vi "Upload info from spreadsheet.vi"(11 "Upload Spreadsheet path":path) -> (3 "Cell Settings Array 1":T1(array[cluster])=[{"Cell Position"=1, "Cell Label"="", "Pixel to measure"=0, "Area (cm^2)"=0.126, "Variable"="", "Variable value"="", "Scan settings in queue"=0}, {"Cell Position"=2, "Cell Label"="", "Pixel to measure"=0, "Area (cm^2)"=0.126, "Variable"="", "Variable value"="", "Scan settings in queue"=0}, {"Cell Position"=3, "Cell Label"="", "Pixel to measure"=0, "Area (cm^2)"=0.126, "Variable"="", "Variable value"="", "Scan settings in queue"=0}, {"Cell Position"=4, "Cell Label"="", "Pixel to measure"=0, "Area (cm^2)"=0.126, "Variable"="", "Variable value"="", "Scan settings in queue"=0}, {"Cell Position"=5, "Cell Label"="", "Pixel to measure"=0, "Area (cm^2)"=0.126, "Variable"="", "Variable value"="", "Scan settings in queue"=0}, {"Cell Position"=6, "Cell Label"="", "Pixel to measure"=0, "Area (cm^2)"=0.126, "Variable"="", "Variable value"="", "Scan settings in queue"=0}, {"Cell Position"=7, "Cell Label"="", "Pixel to measure"=0, "Area (cm^2)"=0.126, "Variable"="", "Variable value"="", "Scan settings in queue"=0}, {"Cell Position"=8, "Cell Label"="", "Pixel to measure"=0, "Area (cm^2)"=0.126, "Variable"="", "Variable value"="", "Scan settings in queue"=0}, {"Cell Position"=9, "Cell Label"="", "Pixel to measure"=0, "Area (cm^2)"=0.126, "Variable"="", "Variable value"="", "Scan settings in queue"=0}, {"Cell Position"=10, "Cell Label"="", "Pixel to measure"=0, "Area (cm^2)"=0.126, "Variable"="", "Variable value"="", "Scan settings in queue"=0}, {"Cell Position"=11, "Cell Label"="", "Pixel to measure"=0, "Area (cm^2)"=0.126, "Variable"="", "Variable value"="", "Scan settings in queue"=0}, {"Cell Position"=12, "Cell Label"="", "Pixel to measure"=0, "Area (cm^2)"=0.126, "Variable"="", "Variable value"="", "Scan settings in queue"=0}, {"Cell Position"=13, "Cell Label"="", "Pixel to measure"=0, "Area (cm^2)"=0.126, "Variable"="", "Variable value"="", "Scan settings in queue"=0}, {"Cell Position"=14, "Cell Label"="", "Pixel to measure"=0, "Area (cm^2)"=0.126, "Variable"="", "Variable value"="", "Scan settings in queue"=0}, {"Cell Position"=15, "Cell Label"="", "Pixel to measure"=0, "Area (cm^2)"=0.126, "Variable"="", "Variable value"="", "Scan settings in queue"=0}, {"Cell Position"=16, "Cell Label"="", "Pixel to measure"=0, "Area (cm^2)"=0.126, "Variable"="", "Variable value"="", "Scan settings in queue"=0}] {"Pixel to measure" items=["All", "1", "2", "3", "4", "5", "6", "7", "8"]})   [LabVIEW 2011]
uses:
  <vilib>/Utility/file.llb/Read From Spreadsheet File (string).vi
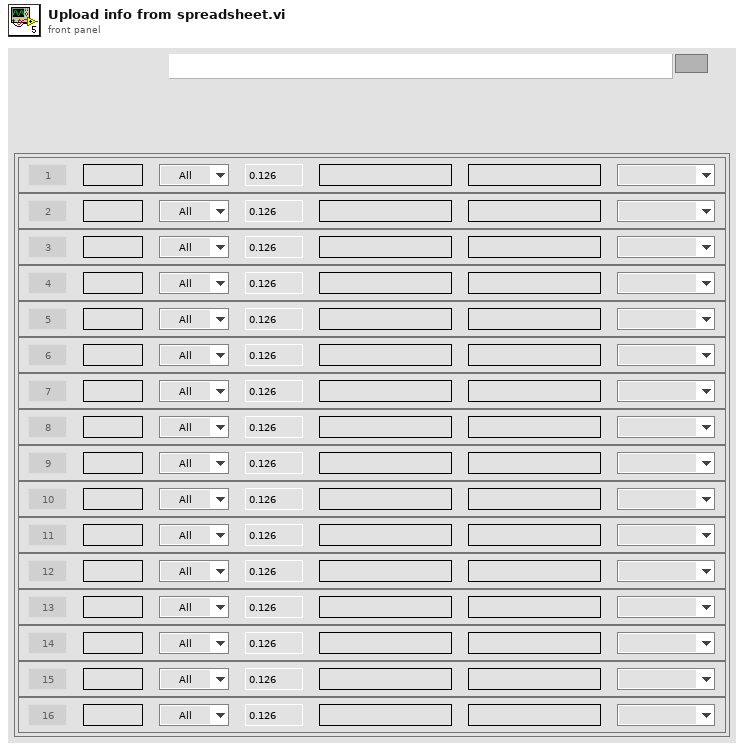
[diagram p1: front panel]
types:
  T1 = cluster{"Cell Position":i32, "Cell Label":string, "Pixel to measure":u16, "Area (cm^2)":dbl, "Variable":string, "Variable value":string, "Scan settings in queue":u16}[]
  T2 = cluster{"Cell Position":i32, "Cell Label":string, "Pixel to measure":u16, "Area (cm^2)":dbl, "Variable":string, "Variable value":string, "Scan settings in queue":u16}
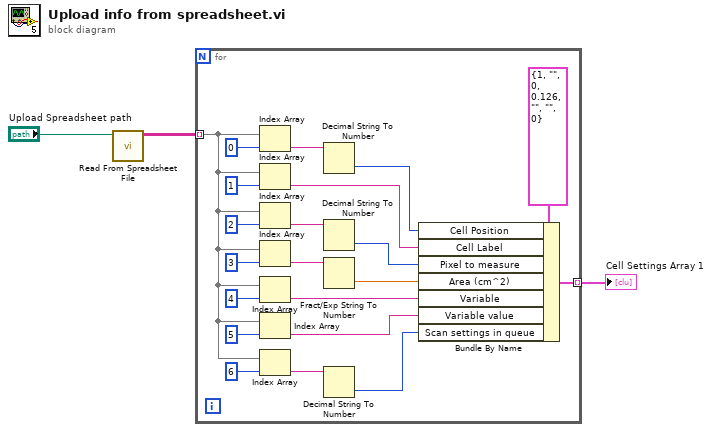
[diagram p0: block diagram]
diagram:
  n1 = call-poly <vilib>:"Read From Spreadsheet File.vi"("file path (dialog if empty)"="Upload Spreadsheet path") -> ("all rows"=w3:string[][])  [unwired: 6 in, 4 out]
  n2 = for {
    tunnel: w3 -> [w24] mode=indexing
    tunnel: [w15] -> w2 mode=indexing
    n3 = Index Array(array=w24, index=0) -> (element=w14:string)
    n4 = Index Array(array=w24, index=1) -> (element=w12:string)
    n5 = Index Array(array=w24, index=2) -> (element=w11:string)
    n6 = Index Array(array=w24, index=3) -> (element=w10:string)
    n7 = Index Array(array=w24, index=4) -> (element=w8:string)
    n8 = Index Array(array=w24, index=5) -> (element=w7:string)
    n9 = Index Array(array=w24, index=6) -> (element=w6:string)
    n10 = Decimal String To Number(string=w14) -> (number=w13:i32)  [unwired: 2 in, 1 out]
    n11 = Decimal String To Number(string=w11) -> (number=w4:i32)  [unwired: 2 in, 1 out]
    n12 = Fract/Exp String To Number(string=w10) -> (number=w9:dbl)  [unwired: 3 in, 1 out]
    n13 = Decimal String To Number(string=w6) -> (number=w5:i32)  [unwired: 2 in, 1 out]
    n14 = Bundle By Name(cluster=T2 {"Cell Position"=1, "Cell Label"="", "Pixel to measure"=0, "Area (cm^2)"=0.126, "Variable"="", "Variable value"="", "Scan settings in queue"=0} ("System Cluster"), "Cell Position"=w13, "Cell Label"=w12, "Pixel to measure"=w4, "Area (cm^2)"=w9, "Variable"=w8, "Variable value"=w7, "Scan settings in queue"=w5) -> (w15:T2)
  }
  "Cell Settings Array 1" <- w2
